vi "Flock_Shared_Get Queue Reference.vi"(8 "Error In":errorcluster, 10 "Enum":T1, 11 "Array":T2) -> (0 "Error Out":errorcluster, 3 "Local Queue out":T3)   [LabVIEW 2014, in "Flock_Shared_Messaging.lvlib"]
uses:
  Flock_Shared_Messaging.lvlib
  <vilib>/NI/AMC/Compatibility/amc_Message Queue.ctl
  ProcessList.ctl
  FGV_Queues.ctl
  Backend/source/VI Source/Dependencies/Keyed Array/KeyedArray.ctl
  Backend/source/VI Source/Dependencies/Keyed Array/Tools_KeyedArray.lvlib
  Backend/source/VI Source/Dependencies/AMC/_SubVIs/TypeDefs/Message.ctl
  Backend/source/VI Source/Dependencies/AMC/AMC.lvlib
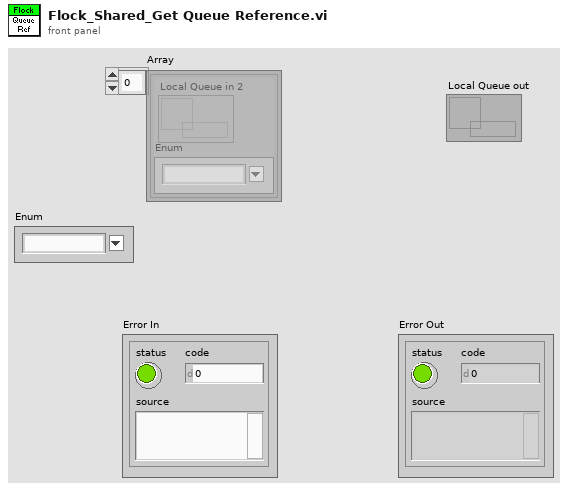
[diagram p1: front panel]
types:
  T1 = typedef "Flock_Shared_Messaging.lvlib/ProcessList.ctl" = string
  T2 = typedef "Flock_Shared_Messaging.lvlib/FGV_Queues.ctl" = cluster{"Local Queue in 2":T3, "Enum":T1}[]
  T3 = typedef "amc_Message Queue.ctl" = refnum<queue>
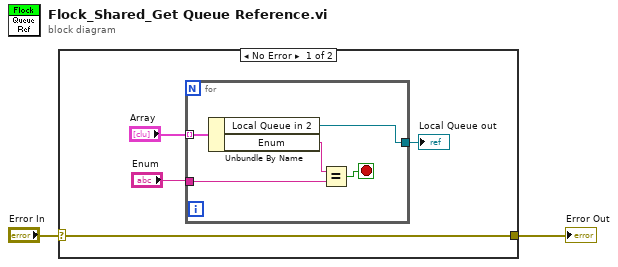
[diagram p0: block diagram]
diagram:
  n1 = case shown="No Error" "Error In" {
    selector: "Error In" -> [w5 w12]
    tunnel: [w5 w12] -> w1
    frame No Error {
      n2 = for {
        tunnel: "Array" -> [w11] mode=indexing
        tunnel: "Enum" -> [w8]
        tunnel: [w7] -> w6
        stop <- w10 stop-if-true
        n3 = Unbundle By Name(w11) -> ("Local Queue in 2"=w7:T3, "Enum"=w9:T1)
        n4 = Equal?(x=w9, y=w8) -> (x = y?=w10:bool)
      }
      "Local Queue out" <- w6
    }
    frame Error {
    }
  }
  "Error Out" <- w1
